vi "observacao.vi"() -> ()   [LabVIEW 2012] (continued)
                    n3074 = call <vilib>:"Draw Flattened Pixmap(6_1).vi"("bit depth(8)"=w3969, "rect"=w3970, "flattened pixmap data"=w3968, "color table"=w3967) -> ("new picture"=→"Image":picture)  [unwired: 5 in]
                    n3075 = call "Acerta_moldura.vi"("fator"=i16 1, "input cluster"=w3970) -> ("Draw Area Size"=w3964:cluster{"Width":u32, "Height":u32})  [unwired: 3 in]
                    n3076 = property on="Image" class="Pict"("Draw Area Size"=w3964) -> ()  [unwired: 2 in, 2 out]
                  }
                }
              }
              frame Enabled {
              }
            }
          }
          frame "All Sky" {
            n3077 = global read "Global_Telescopio.vi" "Tempo Atulização All Sky"() -> (w3972:i16)
            n3078 = call "timepulse_Cam_4.vi"("de quantos segundos"=w3972) -> ("PULSO"=w3973:bool)  [unwired: 2 in]
            n3079 = Or(x="IMAGE 2", y=w3973) -> (x .or. y?=w3974:bool)
            n3080 = case shown="True" w3974 {
              frame False {
              }
              frame True {
                n3081 = stacked-sequence {
                  frame #0 {
                    # "Deixado Propositalmente caso queira colocar uma camera no local do ALL SKY"
                    n3082 = case shown="True" "Case Constant\n(See Context Help) 16" {
                      frame False {
                      }
                      frame True {
                        # "Coloca a moldura na\nImagem"
                        # "Imagen da Cam Setada"
                        n3083 = call "AngeloRTV_Snap.vi"("PortNo"=u16 2) -> ("depth"=w3982:u8, "color table"=w3980:u32[], "rect"=w3983:T11, "flattened image data"=w3981:u8[])  [unwired: 2 in, 1 out]
                        n3084 = call "Acerta_moldura.vi"("fator"=i16 1, "input cluster"=w3983) -> ("Draw Area Size"=w3978:cluster{"Width":u32, "Height":u32})  [unwired: 3 in]
                        "Draw Area 2" <- w3978
                        n3085 = call <vilib>:"Draw Flattened Pixmap(6_1).vi"("bit depth(8)"=w3982, "rect"=w3983, "flattened pixmap data"=w3981, "color table"=w3980) -> ("new picture"=→"Image 2":picture)  [unwired: 5 in]
                        n3086 = property on="Image 2" class="Pict"("Draw Area Size"=w3978) -> ()  [unwired: 2 in, 2 out]
                      }
                    }
                  }
                  frame #1 {
                    # "Fora do ar\n12/02/2009"
                    n3087 = case shown="True" "Case Constant\n(See Context Help) 17" {
                      frame False {
                      }
                      frame True {
                        n3088 = stacked-sequence {
                          seq-local: [w3989 _] -> [_ w3998]
                          frame #0 {
                            n3089 = String To Path(string="C:\\TCSPD_TRABALHO\\IMAGE_TEMP.JPG") -> (path=w3993:path)
                            n3090 = call "URL Get HTTP Document.vi"("follow redirects (T)"="follow redirects (T)", "file path (NAP)"=w3993, "http URL"="http://200.131.64.207/allsky/imagens/allsky_opd.jpg") -> ("error out"=w3988:errorcluster, "file path out"=w3989:path, "header"=→"header":string)  [unwired: 1 in, 5 out]
                            "error out 2" <- w3988
                            n3091 = Unbundle By Name(w3988) -> ("status"=w3987:bool)
                            n3092 = case shown="True" w3987 {
                              frame False {
                              }
                              frame True {
                                n3093 = One Button Dialog(message="Erro durante a aquisição da Imagem do All Sky do site:\n\nhttp://200.131.64.207/allsky/imagens/allsky_opd.jpg") -> ()  [unwired: 1 in, 1 out]
                              }
                            }
                          }
                          frame #1 {
                            (unwired) path "\\\\200.131.64.207/allsky/imagens/allsky_opd.jpg\\" ("path to JPEG file")
                            (unwired) "\\Nasa - Earth From Outer Space.jpg" ("caminho final")
                            # "Isto não está sendo mais usado porémmantive se caso\nseja necessário a manipulação de arquivos com imagem"
                            # "fator de \nredução \nSomente\ninteiros até 6"
                            # "Sem nome de\narquivo ele abre\ncaixa de Diálogo"
                            # "Coloca a moldura na\nImagem"
                            # "Imagen da Cam Setada"
                            n3094 = call "Read JPEG File(6_1).vi"("path to JPEG file"=w3998) -> ("error out"=w4007:errorcluster, "flattened image data"=w4004:u8[], "rect"=w4003:T11, "colorTable"=w4006:u32[], "depth"=w4005:u8)  [unwired: 5 in, 1 out]
                            "error out 3" <- w4007
                            n3095 = String To Path(string="/root/Desktop/Simulador/Nasa - Earth From Outer Space.jpg" ("caminho final")) -> ()  [unwired: 1 out]
                            n3096 = call "Fator_Reducao.vi"("rect"=w4003, "flattened image in"=w4004, "Fator Tamanho"=i16 4) -> ("flattened image out"=w4002:u8[], "area figura x e y"=w3997:cluster{"X Resolution":i32, "Y Resolution":i32})  [unwired: 2 out]
                            n3097 = call "Webcam Flat to Picture.vi"("color table"=w4006, "depth 24/8"=w4005, "error in"=w4007, "rect in"=w4003, "flat image in"=w4002) -> ("error out"=→"error out 4":errorcluster, "picture"=w3996:picture)  [unwired: 2 in, 2 out]
                            n3098 = local write "Draw Area 2"(w3997) -> ()
                            n3099 = property on="Image 2" class="Pict"("Draw Area Size"=w3997) -> ()  [unwired: 2 in, 2 out]
                            n3100 = local write "Image 2"(w3996) -> ()
                            n3101 = call "Cria_path_local.vi"("caminho final"="\\allsky_opd.jpg") -> ()  [unwired: 3 in, 2 out]
                          }
                        }
                      }
                    }
                  }
                }
              }
            }
          }
          frame "Finder" {
            # "Imagem oriunda do\nconector BNC 4"
            n3102 = global read "Global_Telescopio.vi" "Tempo Atulização Cam 3"() -> (w4008:i16)
            n3103 = call "timepulse_Cam_3.vi"("de quantos segundos"=w4008) -> ("PULSO"=w4009:bool)  [unwired: 2 in]
            n3104 = Or(x="IMAGE 4", y=w4009) -> (x .or. y?=w4011:bool)
            n3105 = case shown="True" w4011 {
              frame False {
              }
              frame True {
                n3106 = stacked-sequence {
                  frame #0 {
                    n3107 = call "AngeloRTV_Snap.vi"("PortNo"=u16 3) -> ("depth"=w4017:u8, "color table"=w4015:u32[], "rect"=w4018:T11, "flattened image data"=w4016:u8[])  [unwired: 2 in, 1 out]
                    n3108 = call "Acerta_moldura.vi"("fator"=i16 1, "input cluster"=w4018) -> ("Draw Area Size"=w4012:cluster{"Width":u32, "Height":u32})  [unwired: 3 in]
                    "Draw Area 4" <- w4012
                    n3109 = call <vilib>:"Draw Flattened Pixmap(6_1).vi"("bit depth(8)"=w4017, "rect"=w4018, "flattened pixmap data"=w4016, "color table"=w4015) -> ("new picture"=→"Image 4":picture)  [unwired: 5 in]
                    n3110 = property on="Image 4" class="Pict"("Draw Area Size"=w4012) -> ()  [unwired: 2 in, 2 out]
                  }
                  frame #1 {
                    n3111 = case shown="True" "Case Constant\n(See Context Help) 18" {
                      frame False {
                      }
                      frame True {
                        # "Isto não está sendo mais usado porémmantive se caso\nseja necessário a manipulação de arquivos com imagem"
                        # "fator de \nredução \nSomente\ninteiros até 6"
                        # "Sem nome de\narquivo ele abre\ncaixa de Diálogo"
                        # "Coloca a moldura na\nImagem"
                        # "Imagen da Cam Setada"
                        n3112 = call "Cria_path_local.vi"("caminho final"="\\Nasa - Earth From Outer Space.jpg") -> ("Saida Path inteiro"=w4023:path)  [unwired: 3 in, 1 out]
                        n3113 = call "Read JPEG File(6_1).vi"("path to JPEG file"=w4023) -> ("error out"=w4032:errorcluster, "flattened image data"=w4029:u8[], "rect"=w4028:T11, "colorTable"=w4031:u32[], "depth"=w4030:u8)  [unwired: 5 in, 1 out]
                        n3114 = String To Path(string="/root/Desktop/Simulador/Nasa - Earth From Outer Space.jpg" ("caminho final")) -> ()  [unwired: 1 out]
                        n3115 = call "Fator_Reducao.vi"("rect"=w4028, "flattened image in"=w4029, "Fator Tamanho"=i16 1) -> ("flattened image out"=w4027:u8[], "area figura x e y"=w4021:cluster{"X Resolution":i32, "Y Resolution":i32})  [unwired: 2 out]
                        n3116 = local write "Draw Area 4"(w4021) -> ()
                        n3117 = property on="Image 4" class="Pict"("Draw Area Size"=w4021) -> ()  [unwired: 2 in, 2 out]
                        n3118 = call "Webcam Flat to Picture.vi"("color table"=w4031, "depth 24/8"=w4030, "error in"=w4032, "rect in"=w4028, "flat image in"=w4027) -> ("picture"=w4022:picture)  [unwired: 2 in, 3 out]
                        n3119 = local write "Image 4"(w4022) -> ()
                      }
                    }
                  }
                }
              }
            }
          }
          frame "Telescope" {
            # "Imagem oriunda do\nconector BNC 2"
            n3120 = global read "Global_Telescopio.vi" "Tempo Atulização Cam 1"() -> (w4033:i16)
            n3121 = call "timepulse_Cam_1.vi"("de quantos segundos"=w4033) -> ("PULSO"=w4034:bool)  [unwired: 2 in]
            n3122 = Or(x="IMAGE 3", y=w4034) -> (x .or. y?=w4035:bool)
            n3123 = case shown="True" w4035 {
              frame False {
              }
              frame True {
                n3124 = case shown="True" "Case Constant\n(See Context Help) 19" {
                  frame False {
                  }
                  frame True {
                    n3125 = call "AngeloRTV_Snap.vi"("PortNo"=u16 1) -> ("depth"=w4043:u8, "color table"=w4041:u32[], "rect"=w4044:T11, "flattened image data"=w4042:u8[])  [unwired: 2 in, 1 out]
                    n3126 = call <vilib>:"Draw Flattened Pixmap(6_1).vi"("bit depth(8)"=w4043, "rect"=w4044, "flattened pixmap data"=w4042, "color table"=w4041) -> ("new picture"=→"Image 3":picture)  [unwired: 5 in]
                    n3127 = call "Acerta_moldura.vi"("fator"=i16 1, "input cluster"=w4044) -> ("Draw Area Size"=w4038:cluster{"Width":u32, "Height":u32})  [unwired: 3 in]
                    "Draw Area 3" <- w4038
                    n3128 = property on="Image 3" class="Pict"("Draw Area Size"=w4038) -> ()  [unwired: 2 in, 2 out]
                  }
                }
              }
            }
          }
          frame "Image 3" {
            # "Imagem oriunda do\nconector BNC 3"
            n3129 = global read "Global_Telescopio.vi" "Tempo Atulização Cam 2"() -> (w4046:i16)
            n3130 = call "timepulse_Cam_2.vi"("de quantos segundos"=w4046) -> ("PULSO"=w4047:bool)  [unwired: 2 in]
            n3131 = Or(x="IMAGE 6", y=w4047) -> (x .or. y?=w4049:bool)
            n3132 = case shown="True" w4049 {
              frame False {
              }
              frame True {
                n3133 = call "AngeloRTV_Snap.vi"("PortNo"=u16 2) -> ("depth"=w4055:u8, "color table"=w4053:u32[], "rect"=w4056:T11, "flattened image data"=w4054:u8[])  [unwired: 2 in, 1 out]
                n3134 = call "Acerta_moldura.vi"("fator"=i16 1, "input cluster"=w4056) -> ("Draw Area Size"=w4050:cluster{"Width":u32, "Height":u32})  [unwired: 3 in]
                n3135 = call <vilib>:"Draw Flattened Pixmap(6_1).vi"("bit depth(8)"=w4055, "rect"=w4056, "flattened pixmap data"=w4054, "color table"=w4053) -> ("new picture"=→"Image 3a":picture)  [unwired: 5 in]
                n3136 = property on="Image 3a" class="Pict"("Draw Area Size"=w4050) -> ()  [unwired: 2 in, 2 out]
              }
            }
          }
          frame "Test Only" {
          }
        }
        n3137 = global read "Global_Telescopio.vi" "Caminho camera"() -> (w3957:string)
        n3138 = global read "Global_Telescopio.vi" "stop"() -> (w3958:bool)
        n3139 = call "Greatek.vi"("error in (no error)"="error in (no error)", "Boolean"=w3958, "name or relative path"=w3957, ".NET Refnum in"="PictureBox") -> ("error out"=→"error out 5":errorcluster)  [unwired: 7 in]
      }
      frame #5 {
        w4061 = u16 3 items=["Alarme", "Atencao", "Erro", "Ocupado", "TBD", "LCB", "Trapeira", "Paravento", "DomoRap", "DomoCW", "DomoCCW", "TBD", "Em movimento", "TBD"] ("NomeStatus")
        # "JANELA DE STATUS"
        n3140 = local read "ChkDomeEnable"() -> (w4072:bool)
        n3141 = local read "Flag Stop"() -> (w4067:bool)
        n3142 = case shown="True" w4072 {
          tunnel: [TRUE ("AUX LAMPADA") w4226] -> w4071
          frame False {
          }
          frame True {
            w4232 = u16 3 items=["Alarme", "Atencao", "Erro", "Ocupado", "TBD", "LCB", "Trapeira", "Paravento", "DomoRap", "DomoCW", "DomoCCW", "TBD", "Em movimento", "TBD"] ("NomeStatus")
            n3143 = local read "Dome on Target"() -> (w4229:bool)
            n3144 = local read "statCUP"() -> (w4231:i32)
            n3145 = call "Bit Status CUP.vi"("NomeStatus"=w4232) -> ("StatBit"=w4228:bool)
            n3146 = Equal To 0?(x=w4231) -> (x = 0?=w4230:bool)
            n3147 = Not(x=w4228) -> (.not. x?=w4227:bool)
            n3148 = Compound Arithmetic op=AND(w4230, w4229, w4227) -> (w4226:bool)
          }
        }
        n3149 = case shown="True" w4067 {
          tunnel: [FALSE w4219] -> w4066
          frame False {
          }
          frame True {
            w4223 = u16 3 items=["Alarme", "Atencao", "Erro", "Ocupado", "TBD", "LCB", "Trapeira", "Paravento", "DomoRap", "DomoCW", "DomoCCW", "TBD", "Em movimento", "TBD"] ("NomeStatus")
            n3150 = local read "statCUP"() -> (w4222:i32)
            n3151 = call "Bit Status CUP.vi"("NomeStatus"=w4223) -> ("StatBit"=w4224:bool)
            n3152 = Equal To 0?(x=w4222) -> (x = 0?=w4221:bool)
            n3153 = Not(x=w4224) -> (.not. x?=w4220:bool)
            n3154 = Compound Arithmetic op=AND(w4221, w4220) -> (w4219:bool)
          }
        }
        n3155 = local read "Apontou"() -> (w4079:bool)
        n3156 = local read "BtUtilZenith"() -> (w4087:bool)
        n3157 = local read "BtUtilPark"() -> (w4086:bool)
        n3158 = local read "BtUtilZenith"() -> (w4085:bool)
        n3159 = local read "ECASS"() -> (w4084:bool)
        n3160 = local read "FLAT-FIELD"() -> (w4083:bool)
        n3161 = local read "Flag de erro p/ apagar lampada"() -> (w4062:bool)
        n3162 = call "Bit Status CUP.vi"("NomeStatus"=w4061) -> ("StatBit"=w4060:bool)
        n3163 = Not(x=w4060) -> (.not. x?=w4059:bool)
        n3164 = local read "DEC on Target"() -> (w4073:bool)
        n3165 = local read "RA on Target"() -> (w4074:bool)
        n3166 = Compound Arithmetic op=OR(w4079, w4087, w4086, w4085, w4084, w4083) -> (w4080:bool)
        n3167 = And(x=w4080, y="AUX ABA") -> (x .and. y?=w4082:bool)
        n3168 = Compound Arithmetic op=AND(w4062, w4059) -> (w4058:bool)
        n3169 = case shown="False" w4080 {
          selector: w4080 -> [w4240 _]
          frame False {
            n3170 = Not(x=w4240) -> (.not. x?=w4241:bool)
            n3171 = local write "AUX ABA"(w4241) -> ()
          }
          frame True {
          }
        }
        n3172 = Not(x=w4074) -> (.not. x?=w4075:bool)
        n3173 = Not(x=w4073) -> (.not. x?=w4077:bool)
        n3174 = Not(x=w4071) -> (.not. x?=w4076:bool)
        n3175 = Compound Arithmetic op=AND(w4074, w4073, w4071) -> (w4070:bool)
        n3176 = case shown="True" w4082 {
          selector: w4082 -> [_ w4244]
          frame False {
          }
          frame True {
            # "Liga a câmera de monitoramento"
            # "Ligar a lâmpada pra a câmera"
            n3177 = Not(x=w4244) -> (.not. x?=w4243:bool)
            n3178 = local write "AUX ABA"(w4243) -> ()
            n3179 = local write "Apontou"(w4243) -> ()
            n3180 = local write "AUX LAMPADA"(TRUE ("AUX LAMPADA")) -> ()
            n3181 = local write "Tab Control"(T1."Image 1" ("Tab Control")) -> ()
          }
        }
        n3182 = Compound Arithmetic op=OR(w4075, w4077, w4076) -> (w4078:bool)
        n3183 = And(x=w4070, y="AUX LAMPADA") -> (x .and. y?=w4068:bool)
        n3184 = Or(x=w4068, y=w4066) -> (x .or. y?=w4063:bool)
        n3185 = Or(x=w4063, y=w4058) -> (x .or. y?=w4064:bool)
        n3186 = case shown="True" w4078 {
          selector: w4078 -> [_ w4239]
          frame False {
          }
          frame True {
            n3187 = local write "AUX LAMPADA"(w4239) -> ()
          }
        }
        n3188 = case shown="True" w4064 {
          selector: w4064 -> [_ w4237]
          frame False {
          }
          frame True {
            w4234 = u16 4 items=["ZERO", "AH", "DEC", "TUBO", "CUP"] ("Controlador")
            n3189 = Not(x=w4237) -> (.not. x?=w4233:bool)
            n3190 = local write "AUX LAMPADA"(w4233) -> ()
            n3191 = local write "Flag Stop"(w4233) -> ()
            n3192 = local write "Flag de erro p/ apagar lampada"(w4233) -> ()
            n3193 = local write "Tab Control"(T1."Test Only" ("Tab Control")) -> ()
            n3194 = call "Monta Comando.vi"("Comando"="DESLIGAR", "Dispositivo"="LAMP_CAM", "Controlador"=w4234) -> ()  [unwired: 4 in, 3 out]
          }
        }
        n3195 = global read "Global_Telescopio.vi" "Enable ventilador"() -> (w4065:bool)
        n3196 = Tick Count (ms)() -> (millisecond timer value=w4090:u32)
        n3197 = Subtract(x=w4090, y=w4089) -> (x-y=→"dt":u32)
        n3198 = case shown="True" w4065 {
          frame False {
          }
          frame True {
            w4096 = u16 3 items=["Alarme", "Atencao", "Erro", "Ocupado", "TBD", "LCB", "Trapeira", "Paravento", "DomoRap", "DomoCW", "DomoCCW", "TBD", "Em movimento", "TBD"] ("NomeStatus")
            n3199 = global read "Global_Telescopio.vi" "Hora vent inicial"() -> (w4093:string)
            n3200 = global read "Global_Telescopio.vi" "Hora vent final"() -> (w4092:string)
            n3201 = call "Bit Status TUBO.vi"("NomeStatus"=w4096) -> ("StatBit"=w4095:bool)
            n3202 = call "Comp-HorarioSeg.vi"("Lower limit"=w4093, "Upper limit"=w4092) -> ("In Range?"=w4091:bool)
            n3203 = Not(x=w4095) -> (.not. x?=w4094:bool)
            n3204 = case shown="\"erro_desligar\"" "xxz" {
              tunnel: [w4099 w4123 w4148 w4152 w4165 w4171 w4184] -> w4097
              tunnel: w4091 -> [_ _ w4147 _ w4167 _ w4185]
              tunnel: w4094 -> [w4100 w4124 _ w4151 w4166 w4170 _]
              frame "erro_ligar" {
                n3205 = case shown="True" w4100 {
                  tunnel: ["erro_ligar" w4102] -> w4099
                  frame False {
                  }
                  frame True {
                    w4111 = u16 3 items=["ZERO", "AH", "DEC", "TUBO", "CUP"] ("Controlador")
                    # "super erro"
                    n3206 = call "Monta Comando.vi"("Comando"="LIGAR", "Dispositivo"="VENTILADOR", "Controlador"=w4111) -> ("Resposta"=w4114:string)  [unwired: 4 in, 2 out]
                    n3207 = String Subset(string=w4114, length (rest)=3 ("length (rest)")) -> (substring=w4108:string)  [unwired: 1 in]
                    n3208 = Equal?(x=w4108, y="ACK") -> (x = y?=w4104:bool)
                    n3209 = case shown="False" w4104 {
                      tunnel: [w4115 FALSE] -> w4105
                      tunnel: "erro_ligar" -> [w4116 _]
                      tunnel: [w4116 "espera_desligar"] -> w4103
                      frame False {
                        n3210 = Increment(x="erro lig") -> (x+1=w4117:i32)
                        n3211 = local write "erro lig"(w4117) -> ()
                        n3212 = Greater Or Equal?(x=w4117, y=3) -> (x >= y?=w4115:bool)
                        n3213 = case shown="True" w4115 {
                          frame False {
                          }
                          frame True {
                            w4120 = "Erro de acionamento do ventilador do tubo" ("SYSTEM MESSAGES")
                            n3214 = call "Monta_Mensagem.vi"("Mensagem"=w4120) -> ()  [unwired: 2 in]
                            n3215 = call "Salva_systems_messages.vi"("Mensagem"=w4120) -> ()  [unwired: 5 in]
                          }
                        }
                      }
                      frame True {
                      }
                    }
                    n3216 = Select(t="espera_desligar", s=w4105, f=w4103) -> (s? t:f=w4102:string)
                  }
                }
              }
              frame "erro_desligar" {
                n3217 = case shown="True" w4124 {
                  tunnel: ["erro_desligar" w4126] -> w4123
                  frame False {
                  }
                  frame True {
                    w4136 = u16 3 items=["ZERO", "AH", "DEC", "TUBO", "CUP"] ("Controlador")
                    # "super erro"
                    n3218 = call "Monta Comando.vi"("Comando"="DESLIGAR", "Dispositivo"="VENTILADOR", "Controlador"=w4136) -> ("Resposta"=w4134:string)  [unwired: 4 in, 2 out]
                    n3219 = String Subset(string=w4134, length (rest)=3 ("length (rest)")) -> (substring=w4132:string)  [unwired: 1 in]
                    n3220 = Equal?(x=w4132, y="ACK") -> (x = y?=w4131:bool)
                    n3221 = case shown="False" w4131 {
                      tunnel: [w4139 FALSE] -> w4130
                      tunnel: "erro_desligar" -> [w4140 _]
                      tunnel: [w4140 "aguardando _ligar"] -> w4128
                      frame False {
                        n3222 = Increment(x="erro des") -> (x+1=w4142:i32)
                        n3223 = local write "erro des"(w4142) -> ()
                        n3224 = Greater Or Equal?(x=w4142, y=3) -> (x >= y?=w4139:bool)
                        n3225 = case shown="True" w4139 {
                          frame False {
                          }
                          frame True {
                            w4144 = "Erro de acionamento do ventilador do tubo" ("SYSTEM MESSAGES")
                            n3226 = call "Monta_Mensagem.vi"("Mensagem"=w4144) -> ()  [unwired: 2 in]
                            n3227 = call "Salva_systems_messages.vi"("Mensagem"=w4144) -> ()  [unwired: 5 in]
                          }
                        }
                      }
                      frame True {
                      }
                    }
                    n3228 = Select(t="aguardando _ligar", s=w4130, f=w4128) -> (s? t:f=w4126:string)
                  }
                }
              }
              frame "inicio", Default {
                n3229 = Select(t="ligar", s=w4147, f="desligar") -> (s? t:f=w4148:string)
              }
              frame "ligar" {
                n3230 = case shown="True" w4151 {
                  tunnel: ["ligar" w4155] -> w4152
                  frame False {
                  }
                  frame True {
                    w4162 = u16 3 items=["ZERO", "AH", "DEC", "TUBO", "CUP"] ("Controlador")
                    n3231 = call "Monta Comando.vi"("Comando"="LIGAR", "Dispositivo"="VENTILADOR", "Controlador"=w4162) -> ("Resposta"=w4160:string)  [unwired: 4 in, 2 out]
                    n3232 = String Subset(string=w4160, length (rest)=3 ("length (rest)")) -> (substring=w4158:string)  [unwired: 1 in]
                    n3233 = Equal?(x=w4158, y="ACK") -> (x = y?=w4154:bool)
                    n3234 = Select(t="espera_desligar", s=w4154, f="erro_ligar") -> (s? t:f=w4155:string)
                  }
                }
              }
              frame "espera_desligar" {
                n3235 = case shown="False" w4167 {
                  tunnel: w4166 -> [_ _]
                  tunnel: ["desligar" "espera_desligar"] -> w4165
                  frame False {
                    # "Já ligou mas saiu da faixa e deve desligar"
                  }
                  frame True {
                    # "Já ligou mas está na faixa"
                  }
                }
              }
              frame "desligar" {
                n3236 = case shown="True" w4170 {
                  tunnel: ["desligar" w4173] -> w4171
                  frame False {
                  }
                  frame True {
                    w4181 = u16 3 items=["ZERO", "AH", "DEC", "TUBO", "CUP"] ("Controlador")
                    n3237 = call "Monta Comando.vi"("Comando"="DESLIGAR", "Dispositivo"="VENTILADOR", "Controlador"=w4181) -> ("Resposta"=w4179:string)  [unwired: 4 in, 2 out]
                    n3238 = String Subset(string=w4179, length (rest)=3 ("length (rest)")) -> (substring=w4177:string)  [unwired: 1 in]
                    n3239 = Equal?(x=w4177, y="ACK") -> (x = y?=w4176:bool)
                    n3240 = Select(t="aguardando _ligar", s=w4176, f="erro_desligar") -> (s? t:f=w4173:string)
                  }
                }
              }
              frame "aguardando _ligar" {
                n3241 = case shown="True" w4185 {
                  tunnel: ["aguardando _ligar" "ligar"] -> w4184
                  frame False {
                  }
                  frame True {
                  }
                }
              }
            }
            n3242 = local write "xxz"(w4097) -> ()
          }
        }
        n3243 = stacked-sequence {
          frame #0 {
            n3244 = Get Date/Time String(want seconds? (F)=TRUE ("Boolean")) -> (time string=w4190:string)  [unwired: 2 in, 1 out]
            n3245 = In Range and Coerce(upper limit="16:00:01", x=w4190, lower limit="15:59:59" ("upper limit")) -> (In Range?=w4189:bool)  [unwired: 1 out]
            n3246 = In Range and Coerce(upper limit="17:45:01", x=w4190, lower limit="17:44:59" ("upper limit")) -> (In Range?=w4188:bool)  [unwired: 1 out]
            n3247 = case shown="True" w4188 {
              selector: w4188 -> [_ w4196]
              frame False {
              }
              frame True {
                "Flag desligar" <- w4196
              }
            }
            n3248 = case shown="True" w4189 {
              selector: w4189 -> [_ w4197]
              frame False {
              }
              frame True {
                "Flag ligar" <- w4197
              }
            }
          }
          frame #1 {
            n3249 = local read "Flag ligar"() -> (w4199:bool)
            n3250 = local read "Flag desligar"() -> (w4198:bool)
            n3251 = Or(x=w4199, y=w4198) -> (x .or. y?=w4200:bool)
            n3252 = case shown="True" w4200 {
              tunnel: w4199 -> [_ w4201]
              tunnel: w4198 -> [_ w4203]
              frame False {
              }
              frame True {
                w4207 = u16 3 items=["Alarme", "Atencao", "Erro", "Ocupado", "TBD", "LCB", "Trapeira", "Paravento", "DomoRap", "DomoCW", "DomoCCW", "TBD", "Em movimento", "TBD"] ("NomeStatus")
                n3253 = call "Bit Status TUBO.vi"("NomeStatus"=w4207) -> ("StatBit"=w4206:bool)
                n3254 = Not(x=w4206) -> (.not. x?=w4202:bool)
                n3255 = And(x=w4202, y=w4203) -> (x .and. y?=w4204:bool)
                n3256 = And(x=w4201, y=w4202) -> (x .and. y?=w4205:bool)
                n3257 = case shown="True" w4204 {
                  selector: w4204 -> [_ w4212]
                  frame False {
                  }
                  frame True {
                    w4208 = u16 3 items=["ZERO", "AH", "DEC", "TUBO", "CUP"] ("Controlador")
                    n3258 = Not(x=w4212) -> (.not. x?=w4211:bool)
                    n3259 = local write "Flag desligar"(w4211) -> ()
                    n3260 = call "Monta Comando.vi"("Comando"="DESLIGAR", "Dispositivo"="VENTILADOR", "Controlador"=w4208) -> ()  [unwired: 4 in, 3 out]
                  }
                }
                n3261 = case shown="True" w4205 {
                  selector: w4205 -> [_ w4217]
                  frame False {
                  }
                  frame True {
                    w4215 = u16 3 items=["ZERO", "AH", "DEC", "TUBO", "CUP"] ("Controlador")
                    n3262 = Not(x=w4217) -> (.not. x?=w4216:bool)
                    n3263 = local write "Flag ligar"(w4216) -> ()
                    n3264 = call "Monta Comando.vi"("Comando"="LIGAR", "Dispositivo"="VENTILADOR", "Controlador"=w4215) -> ()  [unwired: 4 in, 3 out]
                  }
                }
              }
            }
          }
        }
      }
    }
    n3265 = Wait Until Next ms Multiple(millisecond multiple=u32 100) -> ()  [unwired: 1 out]
    n3266 = global read "Global_Telescopio.vi" "stop"() -> (w65:bool)
    n3267 = Or(x=w65, y="sair") -> (x .or. y?=w66:bool)
  }
  n3268 = local write "ChkDomeEnable"(TRUE ("ChkDomeEnable")) -> ()
  n3269 = global write "Global_Telescopio.vi" "Default Met"(FALSE ("ChkDomeEnable")) -> ()
  n3270 = Get Date/Time In Seconds() -> (seconds since 1Jan1904=→"alarm Time":timestamp)
  n3271 = property on="Mensage Alarme" class="Str"("Visible"=w16, "Blinking"=TRUE) -> ()  [unwired: 2 in, 2 out]
  n3272 = property on="Setup, Pointing & Guiding" class="TabCtl (strict)"("MultColors"=TRUE ("Allow Multiple Colors")) -> ()  [unwired: 2 in, 2 out]
  n3273 = case shown="True" FALSE {
    tunnel: w47 -> [_ w4246]
    frame False {
    }
    frame True {
      n3274 = Quit LabVIEW(quit? (T)=w4246) -> ()
    }
  }
  "Flag Alarm" <- w16
  "shutterTimeOld" <- 0 ("shutterTimeOld")
  "sendCommandShutter" <- FALSE ("writeShutterLog")
  "timeStatShutterAlert" <- 0 ("timeStatShutterAlert")
